vi "StartConnectionManager.vi"(0 "STOMP in":refnum<class "STOMP.lvclass">, 1 "address":string, 2 "port":u16, 5 "error in (no error)":errorcluster) -> (14 "STOMP out":refnum<class "STOMP.lvclass">, 19 "error out":errorcluster)   [LabVIEW 2017, in "LabVIEW STOMP.lvlib" / "STOMP.lvclass"]
uses:
  STOMP.lvclass
  ConnectionManager.vi
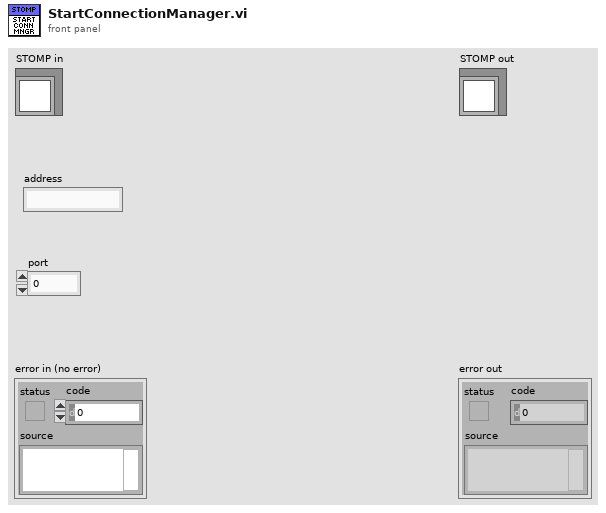
[diagram p1: front panel]
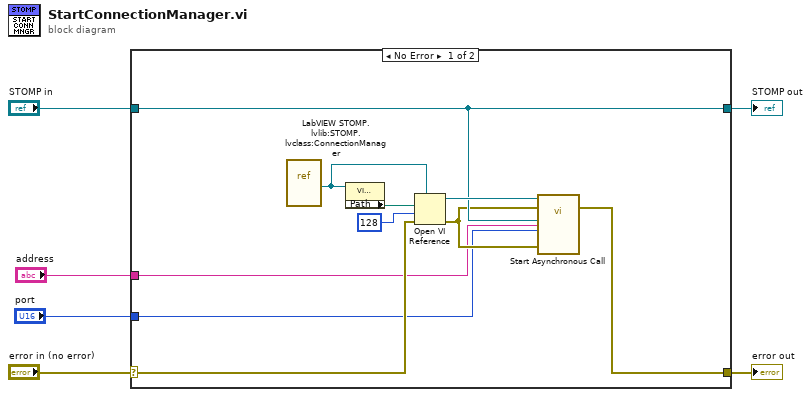
[diagram p0: block diagram]
diagram:
  n1 = case shown="No Error" "error in (no error)" {
    selector: "error in (no error)" -> [w10 w18]
    tunnel: [w9 w18] -> w5
    tunnel: [w12 w17] -> w3
    tunnel: "STOMP in" -> [w12 w17]
    tunnel: "address" -> [w8 _]
    tunnel: "port" -> [w7 _]
    frame No Error {
      n2 = vi-ref "LabVIEW STOMP.lvlib:STOMP.lvclass:ConnectionManager.vi"() -> (w15:refnum<vi>)
      n3 = property class="VI (strict)"(reference=w15) -> ("Path"=w16:path)  [unwired: 1 in, 2 out]
      n4 = Open VI Reference(type specifier VI Refnum (for type only)=w15, vi path=w16, options=128, error in (no error)=w10) -> (vi reference=w13:refnum<vi>, error out=w11:errorcluster)  [unwired: 2 in]
      n5 = call-by-ref "Start Asynchronous Call"(reference=w13, error in=w11, "STOMP In"=w12, "address"=w8, "port"=w7, 5:"error in (no error)"=w11) -> (error out=w9:errorcluster)  [unwired: 15 in, 2 out]
    }
    frame Error {
    }
  }
  "error out" <- w5
  "STOMP out" <- w3
